vi "Get PPMS Helium Level.vi"() -> ()   [LabVIEW 2013]
panel:
  out "SendPPMSCommand Error":i32
  out "PpmsReply":string="79.7,1"
  in  "PpmsCommand":string="LEVEL?"
  in  "Remote":bool=TRUE
  in  "IP Address":string="130.49.180.87"
  # "First Command/Reply"
  # "Instrument Connection"
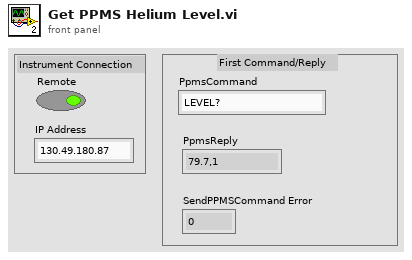
[diagram p1: front panel]
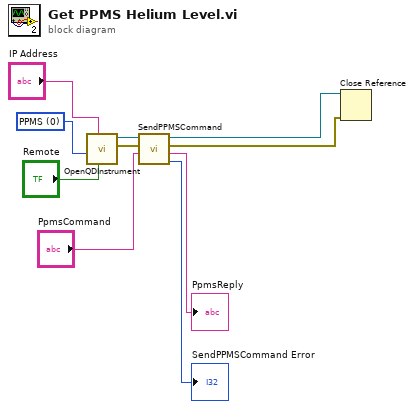
[diagram p0: block diagram]
diagram:
  w6 = 0 items=["PPMS", "VersaLab", "DynaCool", "SVSM"] ("Instrument Type")
  n1 = call "OpenQDInstrument.vi"("Remote"="Remote", "IP Address"="IP Address", "Instrument Type"=w6) -> ("error out"=w9:errorcluster, "Instrument Ref"=w10:refnum<k24>)  [unwired: 5 in]
  n2 = call "SendPPMSCommand.vi"("PpmsCommand"="PpmsCommand", "error in (no error)"=w9, "Instrument Ref In"=w10) -> ("SendPPMSCommand Error"=→"SendPPMSCommand Error":i32, "PpmsReply"=→"PpmsReply":string, "error out"=w1:errorcluster, "Instrument Ref Out"=w2:refnum<k24>)  [unwired: 4 in, 1 out]
  n3 = Close Reference(reference=w2, error in (no error)=w1) -> ()  [unwired: 1 out]
